vi "power conversion.vi"(8 "error in (no error)":errorcluster, 11 "AOTF in":refnum<class "AOTF.lvclass">) -> (0 "error out":errorcluster, 3 "AOTF out":refnum<class "AOTF.lvclass">)   [LabVIEW 2012, in "AOTF.lvclass"]
uses:
  AOTF.lvclass
  AOTF.lvclass/AOTF.ctl
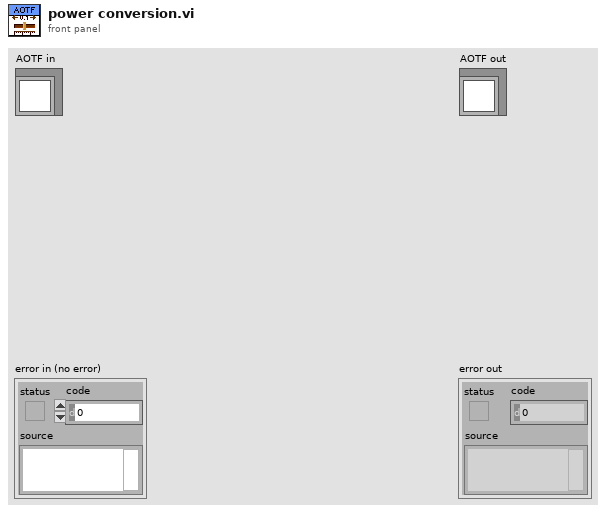
[diagram p1: front panel]
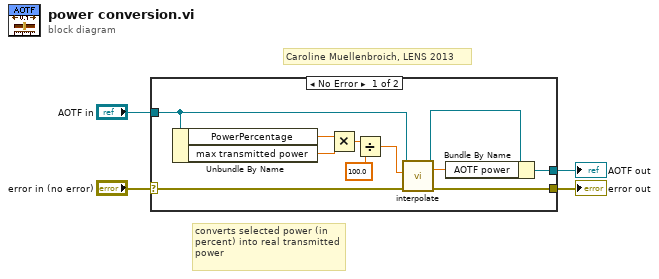
[diagram p0: block diagram]
diagram:
  # "converts selected power (in percent) into real transmitted power"
  # "Caroline Muellenbroich, LENS 2013"
  n1 = case shown="No Error" "error in (no error)" {
    selector: "error in (no error)" -> [w15 w17]
    tunnel: [w14 w17] -> w3
    tunnel: [w5 w16] -> w1
    tunnel: "AOTF in" -> [w13 w16]
    frame No Error {
      n2 = Unbundle By Name(w13) -> ("PowerPercentage"=w12:dbl, "max transmitted power"=w11:dbl)
      n3 = Multiply(x=w12, y=w11) -> (x*y=w10:dbl)
      n4 = Divide(x=w10, y=100.0) -> (x/y=w8:dbl)
      n5 = call-dynamic "interpolate.vi"("error in (no error)"=w15, "element in"=w8, "AOTF in"=w13) -> ("error out"=w14:errorcluster, "element out"=w7:dbl, "AOTF out"=w6:refnum<class "AOTF.lvclass">)  [unwired: 6 in]
      n6 = Bundle By Name(cluster=w6, "AOTF power"=w7) -> (w5:refnum<class "AOTF.lvclass">)
    }
    frame Error {
    }
  }
  "error out" <- w3
  "AOTF out" <- w1
